vi "Update Step Description.vi"(9 "Step Settings":T1, 10 "Step tag":string, 11 "UI Data in":refnum<class "Settings UI.lvclass">) -> (3 "UI Data out":refnum<class "Settings UI.lvclass">)   [LabVIEW 2020, in "Output Sequencer.lvlib" / "Settings UI.lvclass"]
uses:
  Settings UI.lvclass
  Types/Step Settings.ctl
  Settings UI.lvclass/Settings UI.ctl
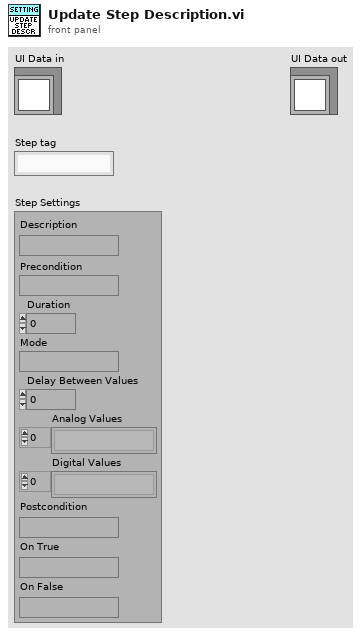
[diagram p1: front panel]
types:
  T1 = typedef "Output Sequencer.lvlib/Settings UI.lvclass/Step Settings.ctl" = cluster{"Description":string, "Precondition":string, "Duration":dbl, "Mode":string, "Delay Between Values":dbl, "Analog Values":string[], "Digital Values":string[], "Postcondition":string, "On True":string, "On False":string}
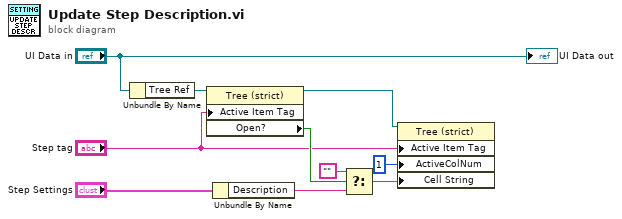
[diagram p0: block diagram]
diagram:
  n1 = Unbundle By Name("UI Data in") -> ("Tree Ref"=w4:refnum<vi>)
  n2 = property class="Tree (strict)"(reference=w4, "Active Item Tag"="Step tag") -> (reference out=w5:refnum<vi>, "Open?"=w6:bool)  [unwired: 1 in, 1 out]
  n3 = Unbundle By Name("Step Settings") -> ("Description"=w9:string)
  n4 = Select(t="", s=w6, f=w9) -> (s? t:f=w10:string)
  n5 = property class="Tree (strict)"(reference=w5, "Active Item Tag"="Step tag", "ActiveColNum"=1 ("Active Cell:Active Column Number"), "Cell String"=w10) -> ()  [unwired: 1 in, 2 out]
  "UI Data out" <- "UI Data in"
